vi "SR830 - Kepco - Hysteresis Measurment - No Noise.vi"() -> ()   [LabVIEW 2016]
uses:
  <vilib>/express/express shared/transition.llb/Dynamic To Waveform Array.vi
  <vilib>/express/express signal manip/GetorSetDDTAttributes/Set DDT Attributes/SetT0.vi
  <vilib>/express/express shared/transition.llb/Waveform Array To Dynamic.vi
  <vilib>/express/express signal manip/GetorSetDDTAttributes/Set DDT Attributes/Set DDT Properties.xnode
panel:
  in  "Zero Field Wait Time (s)":u32=30
  out "Setup Data":T1
  in  "Sample Name":string="test"
  in  "Directory":string="D:\\JDark\\MTJ Cryostat\\test"
  out "Filename Out":path=path "D:/JDark/MTJ Cryostat/test/test-20mT-hysteresis.lvm"
  in  "Accepted Setup":bool
  in  "Verified Setup":bool
  out "TMR":cluster{dbl[], dbl[]}(graph)={[-0.0544, 0.4456, 0.9352, 1.4248, 1.9143999999999999, 2.404, 2.8935999999999997, 3.3832, 3.8728, 4.362399999999999, 4.852, 5.3416, 5.8312, 6.320799999999999, 6.8104000000000005, 7.3, 7.7896, 8.2792, 8.768799999999999, 9.2584, 10.248000000000001, 10.7272, 11.216800000000001, 11.706399999999999, 12.196, 12.685599999999999, 13.1752, 13.6648, 14.154399999999999, 14.644, 15.133600000000001, 15.6232, 16.1128, 16.6024, 17.092, 17.581599999999998, 18.0712, 18.5608, 19.0504, 19.54, 20.0296, 19.519199999999998, 19.0296, 18.54, 18.0504, 17.5608, 17.0712, 16.581599999999998, 16.092, 15.6024, 15.112799999999998, 14.6232, 14.133600000000001, 13.644, 13.154399999999999, 12.6648, 12.1752, 11.685599999999999, 11.196, 10.706399999999999, 10.216800000000001, 9.7272, 9.237599999999999, 8.748000000000001, 7.7584, 7.2791999999999994, 6.7896, 6.3, 5.8104000000000005, 5.320799999999999, 4.8312, 4.3416, 3.8520000000000003, 3.3623999999999996, 2.8728, 2.3832, 1.8935999999999997, 1.4040000000000001, 0.9143999999999999, 0.42480000000000007, -0.06480000000000002, -0.5544, -1.044, -1.5335999999999999, -2.0232, -2.5128, -3.0023999999999997, -3.492, -3.9816, -4.4712, -4.9608, -5.4504, -5.94, -6.4296, -6.919199999999999, -7.4088, -7.8984000000000005, -8.387999999999998, -8.8776, -9.3672, -9.8568, -10.3464, -10.836, -11.3256, -11.815199999999999, -12.3048, -12.7944, -13.283999999999999, -13.7736, -14.2632, -14.7528, -15.7424, -16.2216, -16.711199999999998, -17.2008, -17.6904, -18.18, -18.6696, -19.159200000000002, -19.648799999999998, -20.138399999999997, -19.628, -19.138399999999997, -18.648799999999998, -18.159200000000002, -17.6696, -17.18, -16.6904, -16.2008, -15.711199999999998, -15.221599999999999, -14.732000000000001, -14.2424, -13.2528, -12.7736, -12.283999999999999, -11.7944, -11.3048, -10.815199999999999, -10.3256, -9.836, -9.3464, -8.8568, -8.3672, -7.877599999999999, -7.387999999999999, -6.8984000000000005, -6.4088, -5.919199999999999, -5.4296, -4.94, -4.4504, -3.9608, -3.4711999999999996, -2.9816, -2.492, -2.0023999999999997, -1.5128, -1.0231999999999999, -0.5335999999999999, -0.04400000000000004], [69953790.21982746, 69994462.77777442, 69967718.61112727, 69943886.0679804, 69954151.73827492, 69916400.47914164, 69966503.45277163, 70017098.40182951, 69957853.90222359, 69979684.38822944, 69966894.03478292, 69958273.31269251, 69970597.54758538, 69927091.5685481, 69951274.15493505, 69975111.73394063, 70025342.38913666, 70101179.50987609, 69983374.78232008, 69890957.2826106, 69969758.43611526, 69983374.78232008, 70010101.95320812, 70010550.95864438, 69965649.97392254, 70003932.33277875, 70017895.18756127, 69996084.29346387, 69998589.10374463, 69964854.37679826, 69973057.12818795, 69978454.34335361, 69973491.18977337, 69934851.8795055, 69940590.12561432, 69990307.98671071, 69945129.35499595, 69997734.84194495, 69927452.81109615, 69944305.31098829, 69948411.266759, 69959922.07844894, 69958287.77521215, 70005177.75540388, 69971827.3162728, 69998965.56471586, 70030675.21091811, 69935227.65522334, 69997343.9155331, 69980494.7943649, 69945519.69840819, 70003917.85138094, 69957029.55837137, 70012593.28185017, 70001847.07317972, 69909770.75678013, 69937308.9477036, 69987876.14275324, 69924981.98660928, 69987470.85185637, 69960732.02693424, 69978816.11676958, 69972666.47736529, 69924187.31409012, 69952965.97173885, 69972246.8943031, 69939332.5452715, 69942238.05796859, 69858941.36052282, 69882355.26151025, 70024096.2489493, 70124276.56048097, 69971451.1471442, 69939361.45465657, 69920922.12205227, 69889687.05228348, 69905712.65829201, 69917585.00637151, 70006408.7399148, 70001065.13285743, 69964839.91156349, 69978816.11676958, 69981276.27520046, 69989511.82871358, 69995693.38548763, 69987051.09123293, 69991567.40089324, 69934447.20247924, 69914334.87523946, 69930328.43488088, 69991147.59112982, 69944666.73140821, 70003541.33714098, 69925791.1262778, 69958663.8028221, 69971017.11086768, 69906940.14727889, 69948396.80832255, 69947977.51626554, 69937323.40155673, 69999834.3362578, 69952503.24448285, 69969787.37065852, 69987847.19324781, 69996504.16244982, 69969006.1463901, 69999805.37685895, 69945910.04617715, 69983780.02577896, 69952069.44324002, 69915114.8791537, 69902376.9942027, 69955380.92894632, 69934447.20247924, 69907330.06456648, 69929114.57489035, 69894190.80452518, 69869557.18013413, 69849539.82325777, 69800352.8141219, 69815113.16441435, 69904066.44661842, 69830254.40704262, 69854398.89081328, 69919246.30120051, 69819607.31039546, 69818339.67217934, 69888445.73543541, 69870004.38464876, 69904860.66186896, 69950912.66622883, 69949192.0312033, 69964839.91156349, 69961165.93562299, 69973057.12818795, 69985415.52028471, 69938118.3726788, 69967328.01990989, 69967284.62115493, 69976775.76364617, 69951274.15493505, 69948006.43279776, 69941414.0820846, 69985429.99402861, 70005554.28724681, 69963234.3076816, 69973491.18977337, 69992826.86040007, 69995288.00404988, 69972217.95772569, 69924996.4353677, 69988715.68882897, 70001456.10083497, 69972246.8943031, 69989540.77959612, 69997387.35158546, 69967747.54398352, 69981710.43876189, 69917613.89778097, 69917628.34349464, 70040980.87136921]}
  out "Field (mT)":dbl=-0.04400000000000004
  out "Sample Resistance (Ohms)":dbl=70040980.87136921
  out "Temp (K)":dbl=7.984841572107988 format="%0.3f"
  out "error out":errorcluster
  in  "Step Size (mT)":dbl=0.5 format="%#_13g"
  in  "Field Amplitude (mT)":dbl=2.0 format="%#_13g"
  in  "Rl":dbl=24060.0 format="%#_13g"
  in  "Rp":dbl=1010.0 format="%#_13g"
  in  "error in (no error)":errorcluster
  in  "VISA resource name":refnum<visa-resource-name>="SR830LockIn2"
  # "No final Slashes!"
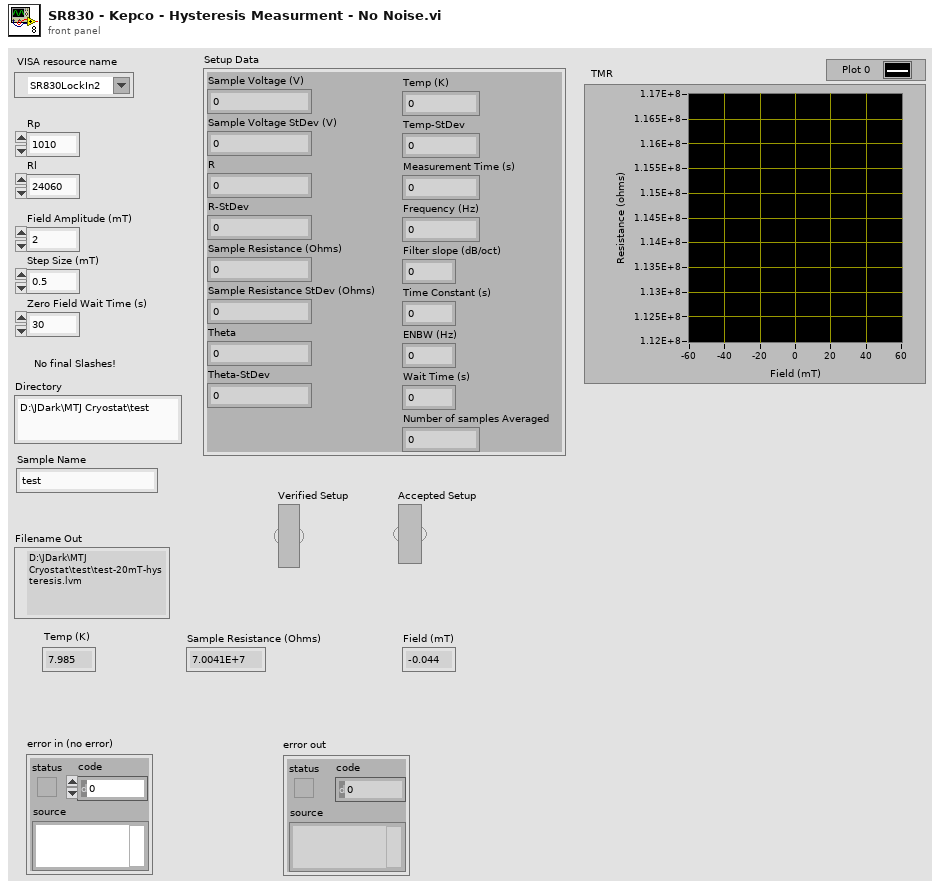
[diagram p1: front panel]
types:
  T1 = cluster{"Sample Voltage (V)":dbl, "Sample Voltage StDev (V)":dbl, "R":dbl, "R-StDev":dbl, "Sample Resistance (Ohms)":dbl, "Sample Resistance StDev (Ohms)":dbl, "Theta":dbl, "Theta-StDev":dbl, "Temp (K)":dbl, "Temp-StDev":dbl, "Measurement Time (s)":dbl, "Frequency (Hz)":dbl, "Filter slope (dB/oct)":dbl, "Time Constant (s)":dbl, "ENBW (Hz)":dbl, "Wait Time (s)":dbl, "Number of samples Averaged":dbl}
  T2 = cluster{"Sample Voltage (V)":dbl, "Sample Voltage StDev (V)":dbl, "R":dbl, "R-StDev":dbl, "Sample Resistance (Ohms)":dbl, "Sample Resistance StDev (Ohms)":dbl, "Theta":dbl, "Theta-StDev":dbl, "Temp (K)":dbl, "Temp-StDev":dbl, "Measurement Time (s)":dbl}
  T3 = cluster{"Sample Voltage (V)":dbl, "Sample Voltage StDev (V)":dbl, "R":dbl, "R-StDev":dbl, "Sample Resistance (Ohms)":dbl, "Sample Resistance StDev (Ohms)":dbl, "Theta":dbl, "Theta-StDev":dbl, "Temp (K)":dbl, "Temp-StDev":dbl, "Measurement Time (s)":dbl, "ReadOut":dbl, "Filter slope (dB/oct)":dbl, "Time Constant (s)":dbl, "ENBW":dbl, "Wait Time (s)":dbl, "Number of samples Averaged":dbl}
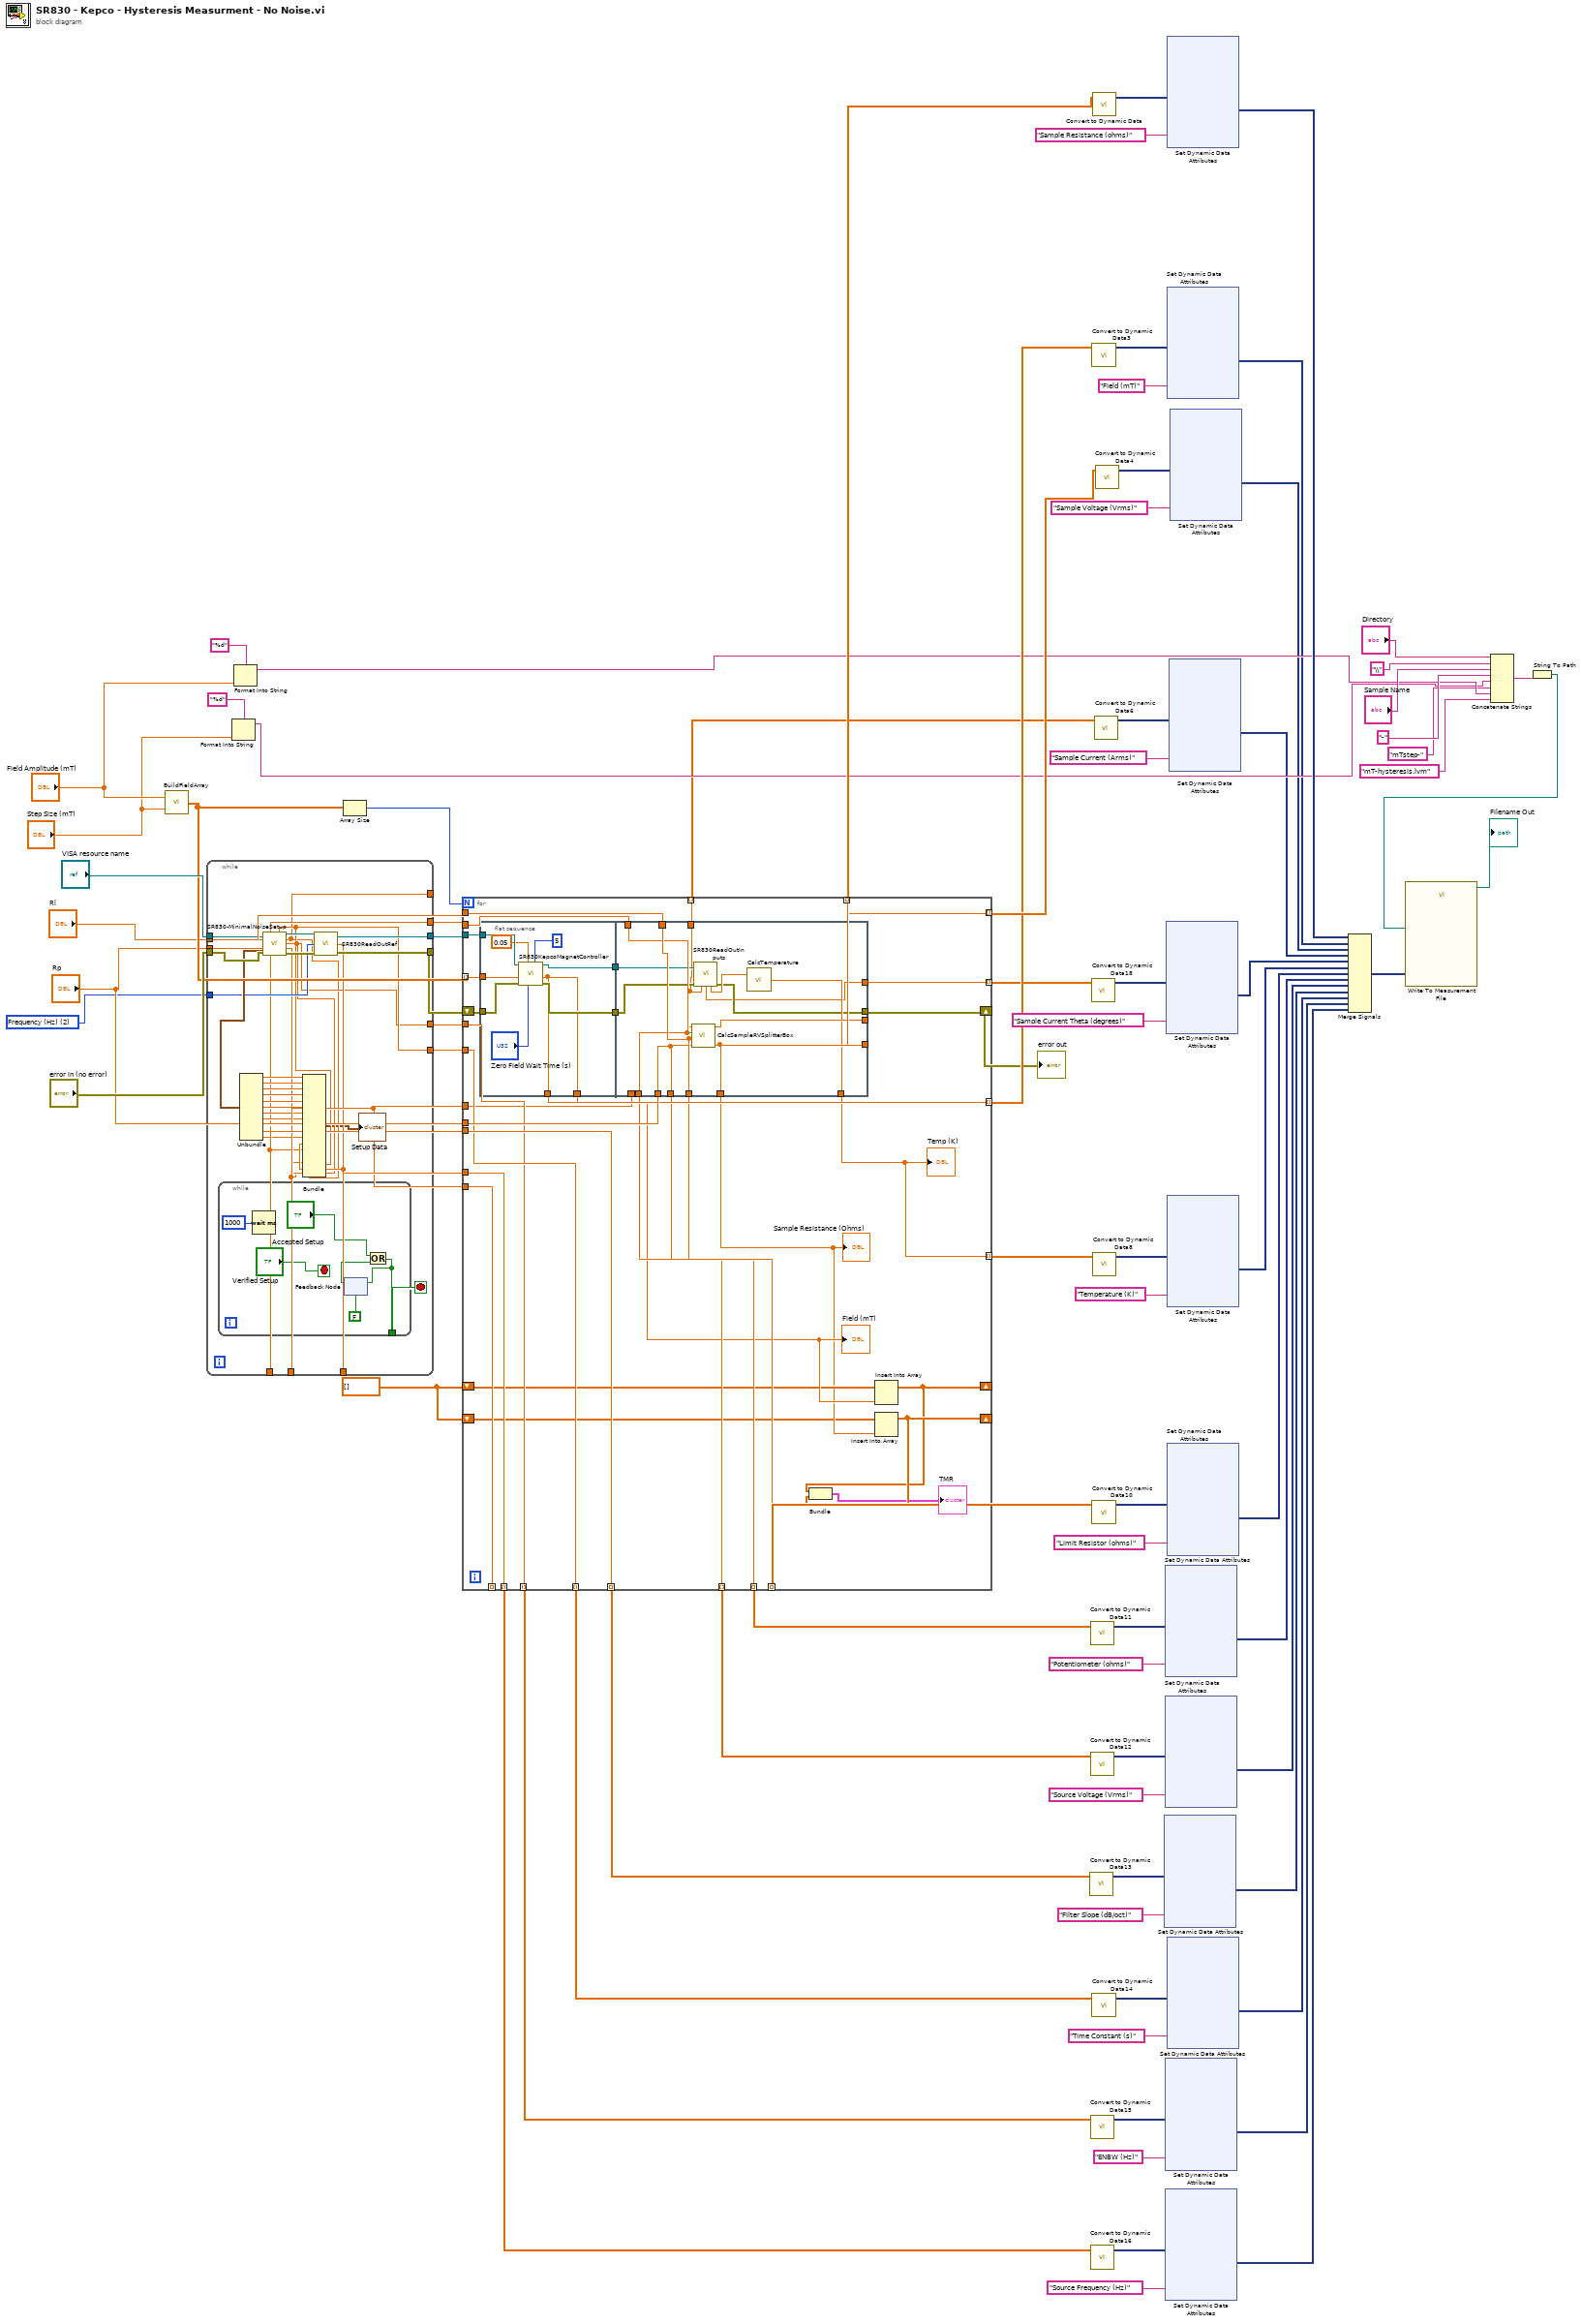
[diagram p0: block diagram]
diagram:
  w31 = u16 2 items=["Voltage Out (Vrms)"=1, "Frequency (Hz)"=2, "Aux Out 1 (VDC)"=3, "Aux Out 2 (VDC)"=4, "Time Constant (s)"=5, "Roll-Off Slope (dB/oct)"=6] ("ReadOut (1: Voltage Amplitude)")
  w32 = dbl[] []
  n1 = call "BuildFieldArray.vi"("Step Size (mT)"="Step Size (mT)", "Field Amplitude (mT)"="Field Amplitude (mT)") -> ("Field Array"=w82:dbl[])
  n2 = while {
    tunnel: "Rp" -> [w111]
    tunnel: [w110] -> w80
    tunnel: "Rl" -> [w109]
    tunnel: [w92] -> w48
    tunnel: [w88] -> _
    tunnel: [w91] -> w46
    tunnel: [w90] -> w44
    tunnel: [w93] -> w42
    tunnel: [w87] -> w37
    tunnel: "error in (no error)" -> [w114]
    tunnel: [w107] -> w33
    tunnel: "VISA resource name" -> [w115]
    tunnel: [w108] -> w38
    tunnel: w31 -> [w94]
    stop <- w89 stop-if-true
    n3 = while {
      tunnel: [w116] -> w89
      stop <- "Verified Setup" stop-if-true
      n4 = Wait (ms)(milliseconds to wait=u32 1000) -> ()  [unwired: 1 out]
      n5 = feedback #1(FALSE ("Accepted Setup")) -> (w117:bool)
      n6 = Or(x="Accepted Setup", y=w117) -> (x .or. y?=w116:bool)
      n7 = feedback-in #1(w116) -> ()
    }
    n8 = call "SR830-MinimalNoiseSetup.vi"("VISA resource name"=w115, "Rl"=w109, "Rp"=w111, "error in (no error)"=w114) -> ("Vs (Vrms)"=w110:dbl, "Time Constant (s)"=w91:dbl, "VISA resource name out"=w113:refnum<visa-resource-name>, "Wait Time (s)"=w88:dbl, "ENBW"=w90:dbl, "Number of samples Averaged"=w87:dbl, "Filter slope (dB/oct)"=w92:dbl, "Setup Data"=w106:T2, "error out"=w112:errorcluster)  [unwired: 3 in]
    n9 = Unbundle(w106) -> ("Sample Voltage (V)"=w105:dbl, "Sample Voltage StDev (V)"=w104:dbl, "R"=w103:dbl, "R-StDev"=w102:dbl, "Sample Resistance (Ohms)"=w101:dbl, "Sample Resistance StDev (Ohms)"=w100:dbl, "Theta"=w99:dbl, "Theta-StDev"=w98:dbl, "Temp (K)"=w97:dbl, "Temp-StDev"=w96:dbl, "Measurement Time (s)"=w95:dbl)
    n10 = call "SR830ReadOutRef.vi"("error in (no error)"=w112, "ReadOut (1: Voltage Amplitude)"=w94, "VISA resource name"=w113) -> ("error out"=w107:errorcluster, "ReadOut"=w93:dbl, "VISA resource name out"=w108:refnum<visa-resource-name>)
    n11 = Bundle("Sample Voltage (V)"=w105, "Sample Voltage StDev (V)"=w104, "R"=w103, "R-StDev"=w102, "Sample Resistance (Ohms)"=w101, "Sample Resistance StDev (Ohms)"=w100, "Theta"=w99, "Theta-StDev"=w98, "Temp (K)"=w97, "Temp-StDev"=w96, "Measurement Time (s)"=w95, "ReadOut"=w93, "Filter slope (dB/oct)"=w92, "Time Constant (s)"=w91, "ENBW"=w90, "Wait Time (s)"=w88, "Number of samples Averaged"=w87) -> (→"Setup Data":T3)  [unwired: 1 in]
  }
  n12 = Format Into String(format string="%d", "Step Size (mT)") -> (resulting string=w16:string)  [unwired: 2 in, 1 out]
  n13 = Format Into String(format string="%d", "Field Amplitude (mT)") -> (resulting string=w18:string)  [unwired: 2 in, 1 out]
  n14 = Array Size(array=w82) -> (size(s)=w83:i32)
  n15 = for {
    N: w83 -> [_]
    tunnel: w82 -> [w152] mode=indexing
    tunnel: "Rp" -> [w151]
    tunnel: "Rl" -> [w150]
    tunnel: w80 -> [w149]
    tunnel: [w148] -> w54 mode=indexing
    tunnel: [w147] -> w53 mode=indexing
    tunnel: [w146] -> w52 mode=indexing
    tunnel: [w145] -> w51 mode=indexing
    tunnel: [w144] -> w50 mode=indexing
    tunnel: [w143] -> w49 mode=indexing
    tunnel: [w142] -> w47 mode=indexing
    tunnel: w48 -> [w142]
    tunnel: w46 -> [w141]
    tunnel: [w141] -> w45 mode=indexing
    tunnel: w44 -> [w140]
    tunnel: [w140] -> w43 mode=indexing
    tunnel: w42 -> [w139]
    tunnel: [w139] -> w41 mode=indexing
    tunnel: w37 -> [w138]
    tunnel: [w138] -> _ mode=indexing
    tunnel: w38 -> [w137]
    tunnel: w37 -> [w136]
    shift-right: [w125] -> w34
    shift-left: w33 -> [w135]
    shift-right: [w127] -> _
    shift-left: w32 -> [w133]
    shift-right: [w130] -> _
    shift-left: w32 -> [w131]
    tunnel: [w124] -> w15 mode=indexing
    tunnel: [w123] -> w14 mode=indexing
    tunnel: [w122] -> w13 mode=indexing
    n16 = flat-sequence {
      tunnel: w152 -> [w161]
      tunnel: [w155] -> w146
      tunnel: w137 -> [w159]
      tunnel: [w158] -> w129
      tunnel: [w157] -> w128
      tunnel: w135 -> [w156]
      tunnel: [w155] -> w134
      tunnel: [w173] -> w147
      tunnel: [w169] -> w148
      tunnel: w151 -> [w171]
      tunnel: w150 -> [w172]
      tunnel: w149 -> [w170]
      tunnel: [w172] -> w145
      tunnel: [w171] -> w144
      tunnel: [w170] -> w143
      tunnel: w136 -> [_]
      tunnel: w129 -> [w165]
      tunnel: w128 -> [w166]
      tunnel: [w169] -> w132
      tunnel: [w167] -> w124
      tunnel: [w164] -> w125
      tunnel: [w163] -> w123
      tunnel: [w162] -> w122
      frame #0 {
        n17 = call "SR830KepcoMagnetController.vi"("Field dwell time (ms)"=u32 5, "Zero Field Wait (s)"="Zero Field Wait Time (s)", "Field Step size (mT)"=0.05, "error in (no error)"=w156, "Target Field (mT)"=w161, "VISA resource name"=w159) -> ("error out"=w158:errorcluster, "Final Field (mT)"=w155:dbl, "VISA resource name out"=w157:refnum<visa-resource-name>)  [unwired: 2 in, 1 out]
      }
      frame #1 {
        n18 = call "SR830ReadOutInputs.vi"("VISA resource name"=w166, "error in (no error)"=w165) -> ("R"=w162:dbl, "Theta"=w163:dbl, "Aux In 1"=w168:dbl, "error out"=w164:errorcluster)  [unwired: 9 in, 1 out]
        n19 = call "CalcSampleRVSplitterBox.vi"("Rp"=w171, "Rl"=w172, "Source Voltage (V)"=w170, "Sample Current (A)"=w162) -> ("Sample Resistance (Ohms)"=w169:dbl, "Sample Voltage (V)"=w173:dbl)  [unwired: 6 in]
        n20 = call "CalcTemperature.vi"("Temp Voltage (V)"=w168) -> ("Temperature (K)"=w167:dbl)  [unwired: 1 in]
      }
    }
    n21 = Insert Into Array(array=w133, new element=w134) -> (w127:dbl[])  [unwired: 1 in]
    n22 = Insert Into Array(array=w131, new element=w132) -> (w130:dbl[])  [unwired: 1 in]
    n23 = Bundle(w127, w130) -> (→"TMR":cluster{dbl[], dbl[]})  [unwired: 1 in]
    "Temp (K)" <- w124
    "Sample Resistance (Ohms)" <- w132
    "Field (mT)" <- w134
  }
  "error out" <- w34
  n24 = call "Convert to Dynamic Data13"("Array"=w47) -> ("Dynamic Data Type"=w62:dynamicdata)  [unwired: 3 in]
  n25 = call "Convert to Dynamic Data11"("Array"=w50) -> ("Dynamic Data Type"=w66:dynamicdata)  [unwired: 3 in]
  n26 = call "Convert to Dynamic Data12"("Array"=w49) -> ("Dynamic Data Type"=w64:dynamicdata)  [unwired: 3 in]
  n27 = call "Convert to Dynamic Data15"("Array"=w43) -> ("Dynamic Data Type"=w58:dynamicdata)  [unwired: 3 in]
  n28 = call "Convert to Dynamic Data16"("Array"=w41) -> ("Dynamic Data Type"=w56:dynamicdata)  [unwired: 3 in]
  n29 = call "Convert to Dynamic Data18"("Array"=w14) -> ("Dynamic Data Type"=w36:dynamicdata)  [unwired: 3 in]
  n30 = call "Convert to Dynamic Data3"("Array"=w52) -> ("Dynamic Data Type"=w76:dynamicdata)  [unwired: 3 in]
  n31 = call "Convert to Dynamic Data10"("Array"=w51) -> ("Dynamic Data Type"=w68:dynamicdata)  [unwired: 3 in]
  n32 = call "Convert to Dynamic Data14"("Array"=w45) -> ("Dynamic Data Type"=w60:dynamicdata)  [unwired: 3 in]
  n33 = call "Convert to Dynamic Data"("Array"=w54) -> ("Dynamic Data Type"=w79:dynamicdata)  [unwired: 3 in]
  n34 = call "Convert to Dynamic Data8"("Array"=w15) -> ("Dynamic Data Type"=w70:dynamicdata)  [unwired: 3 in]
  n35 = call "Convert to Dynamic Data6"("Array"=w13) -> ("Dynamic Data Type"=w72:dynamicdata)  [unwired: 3 in]
  n36 = call "Convert to Dynamic Data4"("Array"=w53) -> ("Dynamic Data Type"=w74:dynamicdata)  [unwired: 3 in]
  n37 = xnode "Set Dynamic Data Attributes"("Signals In"=w62, "Signal Name"="Filter Slope (dB/oct)") -> ("Signals Out"=w4:dynamicdata)  [unwired: 2 in, 1 out]
  n38 = xnode "Set Dynamic Data Attributes"("Signals In"=w66, "Signal Name"="Potentiometer (ohms)") -> ("Signals Out"=w6:dynamicdata)  [unwired: 2 in, 1 out]
  n39 = xnode "Set Dynamic Data Attributes"("Signals In"=w64, "Signal Name"="Source Voltage (Vrms)") -> ("Signals Out"=w5:dynamicdata)  [unwired: 2 in, 1 out]
  n40 = xnode "Set Dynamic Data Attributes"("Signals In"=w58, "Signal Name"="ENBW (Hz)") -> ("Signals Out"=w2:dynamicdata)  [unwired: 2 in, 1 out]
  n41 = xnode "Set Dynamic Data Attributes"("Signals In"=w56, "Signal Name"="Source Frequency (Hz)") -> ("Signals Out"=w1:dynamicdata)  [unwired: 2 in, 1 out]
  n42 = xnode "Set Dynamic Data Attributes"("Signals In"=w36, "Signal Name"="Sample Current Theta (degrees)") -> ("Signals Out"=w9:dynamicdata)  [unwired: 2 in, 1 out]
  n43 = xnode "Set Dynamic Data Attributes"("Signals In"=w76, "Signal Name"="Field (mT)") -> ("Signals Out"=w12:dynamicdata)  [unwired: 2 in, 1 out]
  n44 = xnode "Set Dynamic Data Attributes"("Signals In"=w68, "Signal Name"="Limit Resistor (ohms)") -> ("Signals Out"=w7:dynamicdata)  [unwired: 2 in, 1 out]
  n45 = xnode "Set Dynamic Data Attributes"("Signals In"=w60, "Signal Name"="Time Constant (s)") -> ("Signals Out"=w3:dynamicdata)  [unwired: 2 in, 1 out]
  n46 = xnode "Set Dynamic Data Attributes"("Signals In"=w79, "Signal Name"="Sample Resistance (ohms)") -> ("Signals Out"=w39:dynamicdata)  [unwired: 2 in, 1 out]
  n47 = xnode "Set Dynamic Data Attributes"("Signals In"=w70, "Signal Name"="Temperature (K)") -> ("Signals Out"=w8:dynamicdata)  [unwired: 2 in, 1 out]
  n48 = xnode "Set Dynamic Data Attributes"("Signals In"=w72, "Signal Name"="Sample Current (Arms)") -> ("Signals Out"=w10:dynamicdata)  [unwired: 2 in, 1 out]
  n49 = xnode "Set Dynamic Data Attributes"("Signals In"=w74, "Signal Name"="Sample Voltage (Vrms)") -> ("Signals Out"=w11:dynamicdata)  [unwired: 2 in, 1 out]
  n50 = Merge Signals(w39, w12, w11, w10, w9, w8, w7, w6, w5, w4, w3, w2, w1) -> (w40:dynamicdata)
  n51 = Concatenate Strings("Directory", "\\" ("Sample 2"), "Sample Name", "-" ("Sample 2"), w16, "mTstep-" ("Sample 2"), w18, "mT-hysteresis.lvm" ("Sample 2")) -> (w23:string)
  n52 = String To Path(string=w23) -> (path=w22:path)
  n53 = call "Write To Measurement File"("Signals"=w40, "Filename"=w22) -> ("Filename Out"=→"Filename Out":path)  [unwired: 15 in, 2 out]
